vi "dimetix demo.vi"() -> ()   [LabVIEW 2016]
uses:
  message box enable.vi
  <vilib>/Instr/_visa.llb/VISA Configure Serial Port (Instr).vi
panel:
  in  "parity (0:none)":enum16{"None", "Odd", "Even", "Mark", "Space"}(ring)=enum."Even"
  in  "data bits (8) 2":u16=7 min=5 max=8 step=1
  in  "baud rate (9600)":u32=19200
  in  "laser read command":string="s0h"
  out "Numeric":dbl format="%#.3g"
  in  "RS232 \nTIMEOUT":i32=1000
  in  "SERIAL PORT 1":u16(ring) caption="SERIAL PORT" items=["COM1  (ASRL1  )", "COM3  (ASRL3  )", "COM15 (ASRL15  )", "", ""]
  out "READ BUFFER":string
  out "RTN CNT":u32
  out "ERROR WARN":bool caption="ERROR"
  in  "READ":bool
  in  "stop vi":bool
  in  "joint cluster PIPE01":T1(array[cluster]) {"length" format="%.2f"}
  in  "step 1\ninitalize serial":bool
  out "command sent":string="s0c\r\n"
  out "after substring":string="00001117\r\n"
  out "error out":errorcluster
  in  "DEFAULT":T2={"version"="v 1.0.1", "digitally download dir"=path "C:/Documents and Settings/All Users/Application Data/digitally/data", "data Xport path"=path "C:/Program Files/Unitronics/Unitronics DataXport/DataXport.exe", "HTML Save Path"=path "C:/Documents and Settings/All Users/Application Data/digitally/data", "UNIT LABEL"="FEET / TENTHS", "Company name"="Laser-View Technologies"}
  out "FILE SAVED ONCE":bool
  in  "INPUT CLUSTER":T3={"READ DIRECTION"=TRUE, "MEASUREMENT SOURCE"=0, "GROUP ANALYSIS METHOD"=0, "units"=2, "SERIAL PORT 1"=0, "SERIAL PORT 2"=1, "SERIAL PORT 3"=0, "GROUP SIZE"=1, "OFFSET- 2 laser"=0.0, "ACTUAL MEAUSURE"=0.0, "MEASURE SPEED"=2, "DISTANCE DELTA \nFOR FAST MODE (mm)"=1.0, "laser 1 OFFSET"=1.0, "laser 2 OFFSET"=0.0, "ENABLE SENSOR A"=TRUE, "ENABLE SENSOR B"=TRUE, "ENABLE SENSOR C"=TRUE, "PORT TIMEOUT (msec)"=300, "PASSWORD"="", "ENABLE ON-SCREEN\nKEYBOARD"=TRUE, "version"="", "BUFER LENGTH"=100, "TRIGGER DELAY (msec)"=100, "DATA LOG  FILE DIR"=path "C:/Documents and Settings/All Users/Application Data/PMS200", "MEASUREMENT TYPE"=0, "ENABLE DATA LOG"=FALSE, " LIMITS SENSOR 1"={"Upper tol"=4.3, "Lower tol"=0.0, "STATUS"=FALSE, "Boolean"=FALSE}, " LIMITS SENSOR 2"={"Upper tol"=0.0, "Lower tol"=0.0, "STATUS"=FALSE, "Boolean"=FALSE}, " CALC LIMITS"={"Upper tol"=0.0, "Lower tol"=0.0, "STATUS"=FALSE, "Boolean"=FALSE}, "LASER 2\n ENABLE"=FALSE, "LASER 1 \nENABLE"=TRUE, "BAUD RATE"=1, "PARITY"=2, "DATA BITS"=0, "TRIGGER OPERATION"=0, "TRIGGER LENGTH (sec)"=15.0, "BUFFER METHOD"=0, "DATA LOG METHOD"=0, "LASER 2"=TRUE, "LASER 1"=TRUE, "ACTUAL LASER 2"=0.0, "ACTUAL LASER 1"=0.0, "TWO LASER\n CALIBRATE"=0.0, "OFFSET- TWO LASER 2"=5.0, "Part identification"="100", "JOB ID"="FDFDF", "Operator"="5.5", "Notes"="5.5", "SIZE"="5.5", "WEIGHT"="100", "serial #"=101, "Company name"="BBBB", "LANGUAGE"=0, "LASER \nOFFSET THREADS OFF"=1.0, "LASER \nOFFSET THREADS ON"=1.0, "THREADS ON/OFF"=2, "OPERATION  "=0} {"OPERATION" items=["DRILL SITE- NO S/N", "PIPE YARD- INCLUDE S/N"]; "THREADS ON/OFF" items=["THREADS OFF", "THREADS ON"]; "LASER \nOFFSET THREADS ON" format="%.2f"; "LASER \nOFFSET THREADS OFF" format="%.2f"; "LANGUAGE" items=["ENGLISH", "SPANISH"]; "OFFSET- TWO LASER 2" format="%.2f"; "TWO LASER\n CALIBRATE" format="%.2f"; "ACTUAL LASER 1" format="%.2f"; "ACTUAL LASER 2" format="%.2f"; "DATA LOG METHOD" items=["CONTINUOUS", "TRIGGER SINGLE SHOT", "TRIGGER START/STOP"]; "BUFFER METHOD" items=["BUFFER IN MEMORY", "WRITE IMMEDIATELY"]; "TRIGGER LENGTH (sec)" format="%.1f"; "TRIGGER OPERATION" items=["CLICK START/STOP", "TIMED"]; "DATA BITS" items=["7 (LASER FACTORY DEFAULT", "8", "EVEN"]; "PARITY" items=["NONE", "ODD", "EVEN"]; "BAUD RATE" items=["9600", "19200", "38400", "57600", "115200"]; "CALC LIMITS"."Lower tol" format="%.3f"; "CALC LIMITS"."Upper tol" format="%.3f"; "LIMITS SENSOR 2"."Lower tol" format="%.3f"; "LIMITS SENSOR 2"."Upper tol" format="%.3f"; "LIMITS SENSOR 1"."Lower tol" format="%.3f"; "LIMITS SENSOR 1"."Upper tol" format="%.3f"; "MEASUREMENT TYPE" items=["DISTANCE ", "DIMENSION- SINGLE LASER", "DIMENSION- TWO LASERS DIFFERENTIAL", "DISTANCE DELTA- TWO LASERS"]; "laser 2 OFFSET" format="%.2f"; "laser 1 OFFSET" format="%.2f"; "DISTANCE DELTA \nFOR FAST MODE (mm)" format="%.2f"; "MEASURE SPEED" items=["STANDARD", "FAST"]; "ACTUAL MEAUSURE" format="%.2f"; "OFFSET- 2 laser" format="%.2f"; "GROUP SIZE" min=1; "SERIAL PORT 3" items=["COM1  (ASRL1  )", "COM4 (ASRL4  )", "COM8  (ASRL8  )", "COM9  (ASRL9  )", "", "", ""]; "SERIAL PORT 2" items=["COM1  (ASRL1  )", "COM4 (ASRL4  )", "COM8  (ASRL8  )", "COM9  (ASRL9  )", "", "", ""]; "SERIAL PORT 1" items=["COM1  (ASRL1  )", "COM4 (ASRL4  )", "COM8  (ASRL8  )", "COM9  (ASRL9  )", "", "", ""]; "units" items=["mm", "inch"]; "GROUP ANALYSIS METHOD" items=["mean", "median"]; "MEASUREMENT SOURCE" items=["LIVE", "EMULATE"]}
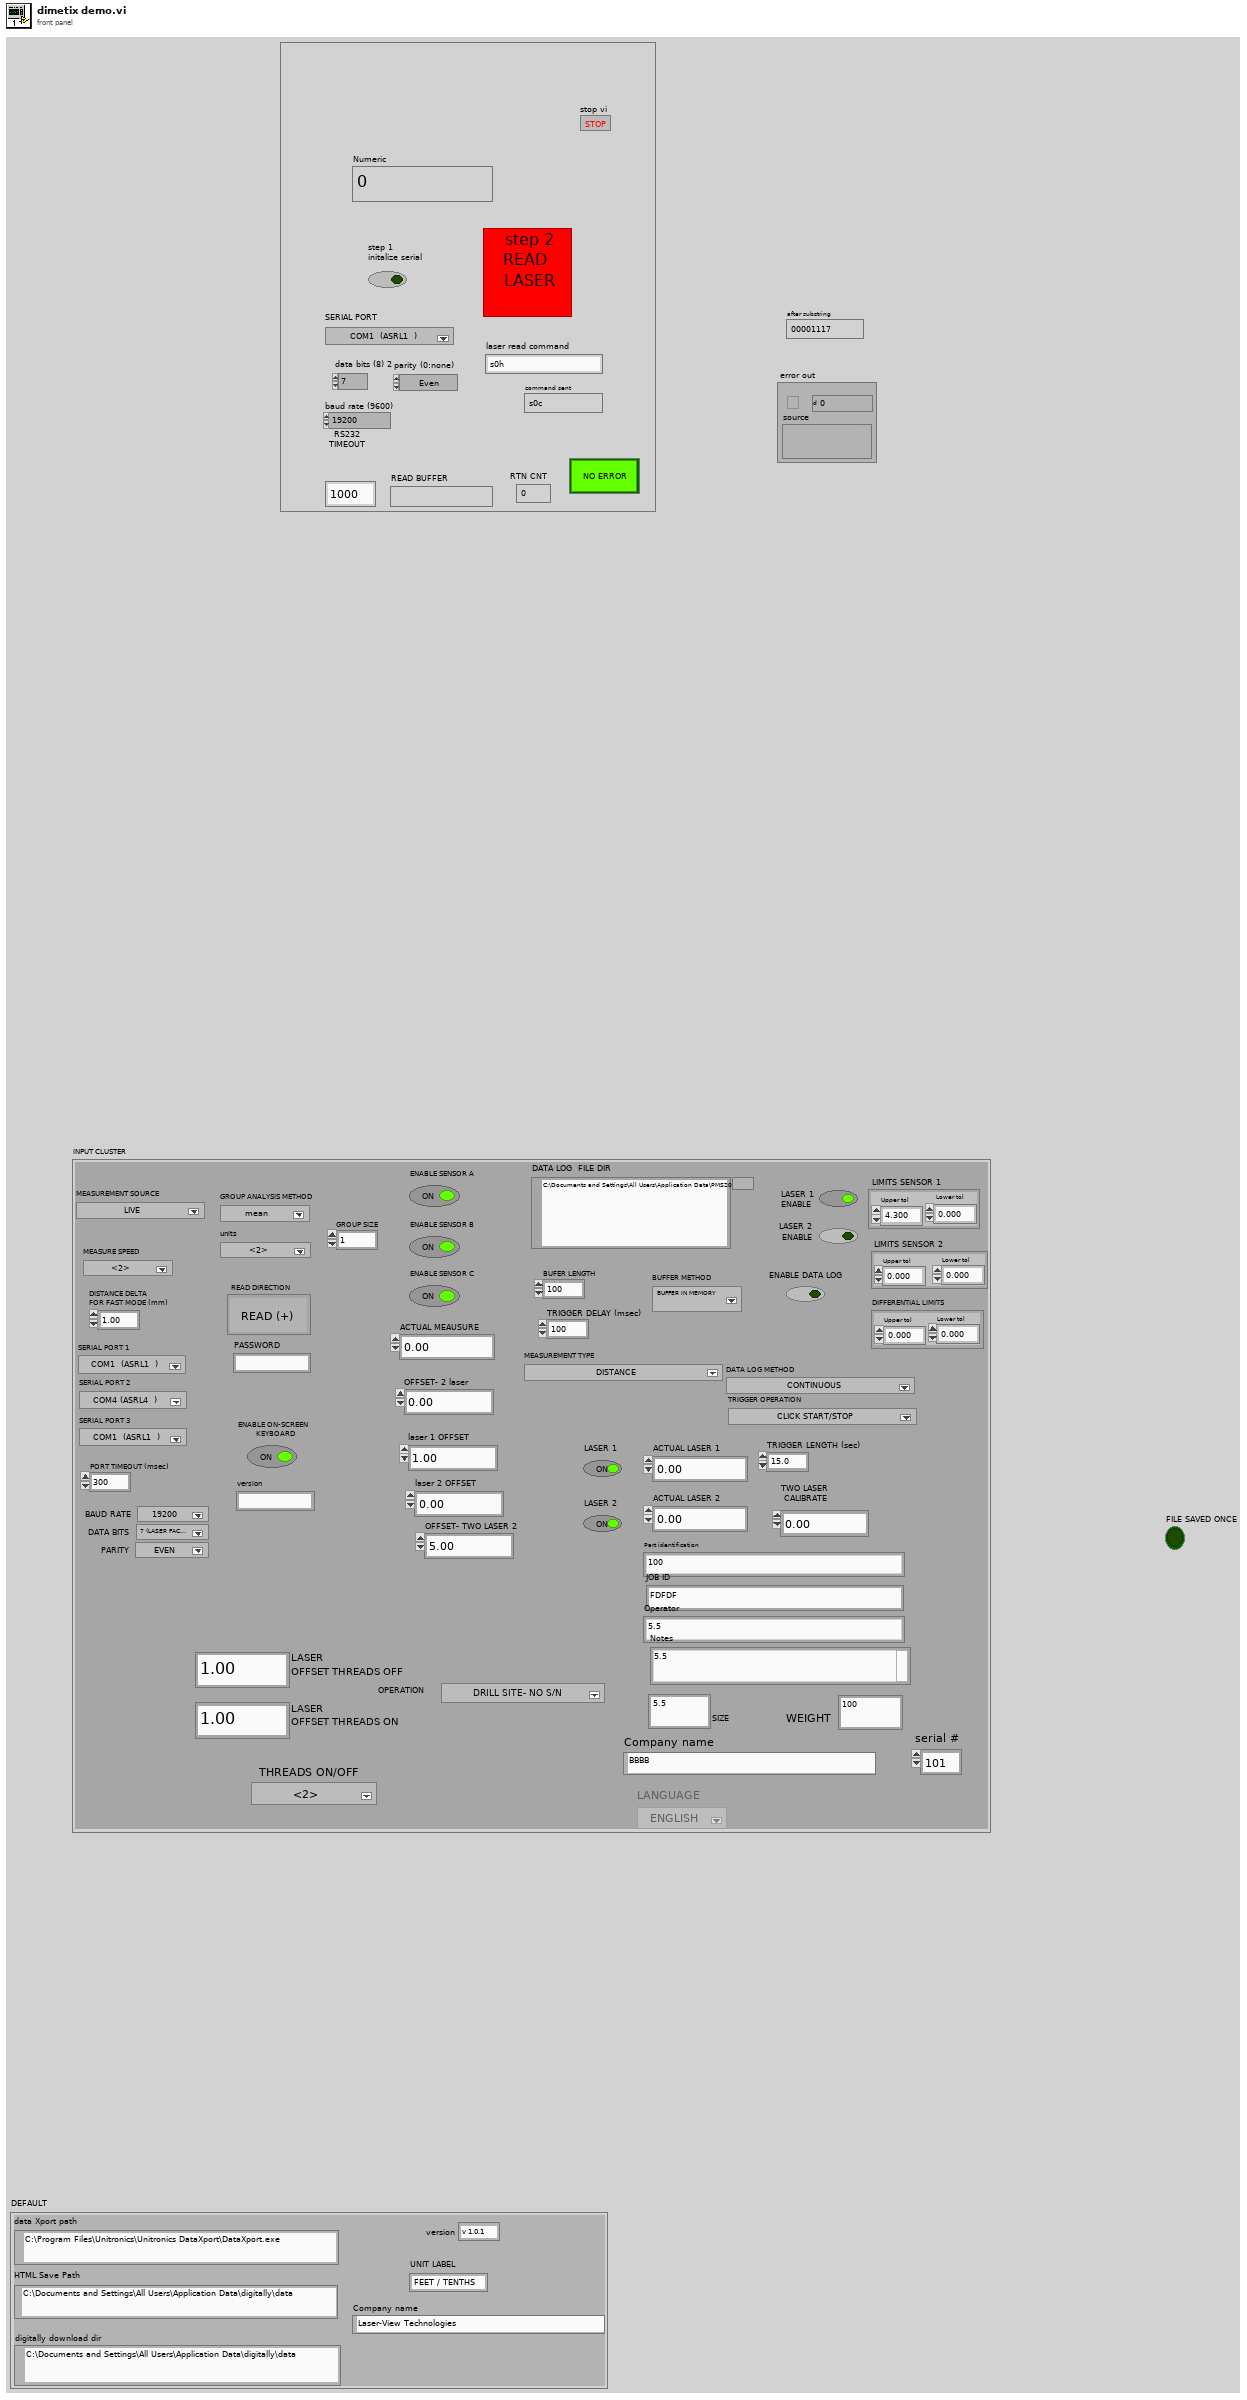
[diagram p1: front panel]
types:
  T1 = cluster{"joint":i32, "length":dbl, "s/n":string}[]
  T2 = cluster{"version":string, "digitally download dir":path, "data Xport path":path, "HTML Save Path":path, "UNIT LABEL":string, "Company name":string}
  T3 = cluster{"READ DIRECTION":bool, "MEASUREMENT SOURCE":u16, "GROUP ANALYSIS METHOD":u16, "units":u16, "SERIAL PORT 1":u16, "SERIAL PORT 2":u16, "SERIAL PORT 3":u16, "GROUP SIZE":i32, "OFFSET- 2 laser":dbl, "ACTUAL MEAUSURE":dbl, "MEASURE SPEED":u16, "DISTANCE DELTA \nFOR FAST MODE (mm)":dbl, "laser 1 OFFSET":dbl, "laser 2 OFFSET":dbl, "ENABLE SENSOR A":bool, "ENABLE SENSOR B":bool, "ENABLE SENSOR C":bool, "PORT TIMEOUT (msec)":i32, "PASSWORD":string, "ENABLE ON-SCREEN\nKEYBOARD":bool, "version":string, "BUFER LENGTH":i32, "TRIGGER DELAY (msec)":i32, "DATA LOG  FILE DIR":path, "MEASUREMENT TYPE":u16, "ENABLE DATA LOG":bool, " LIMITS SENSOR 1":cluster{"Upper tol":dbl, "Lower tol":dbl, "STATUS":bool, "Boolean":bool}, " LIMITS SENSOR 2":cluster{"Upper tol":dbl, "Lower tol":dbl, "STATUS":bool, "Boolean":bool}, " CALC LIMITS":cluster{"Upper tol":dbl, "Lower tol":dbl, "STATUS":bool, "Boolean":bool}, "LASER 2\n ENABLE":bool, "LASER 1 \nENABLE":bool, "BAUD RATE":u16, "PARITY":u16, "DATA BITS":u16, "TRIGGER OPERATION":u16, "TRIGGER LENGTH (sec)":dbl, "BUFFER METHOD":u16, "DATA LOG METHOD":u16, "LASER 2":bool, "LASER 1":bool, "ACTUAL LASER 2":dbl, "ACTUAL LASER 1":dbl, "TWO LASER\n CALIBRATE":dbl, "OFFSET- TWO LASER 2":dbl, "Part identification":string, "JOB ID":string, "Operator":string, "Notes":string, "SIZE":string, "WEIGHT":string, "serial #":i32, "Company name":string, "LANGUAGE":u16, "LASER \nOFFSET THREADS OFF":dbl, "LASER \nOFFSET THREADS ON":dbl, "THREADS ON/OFF":u16, "OPERATION  ":u16}
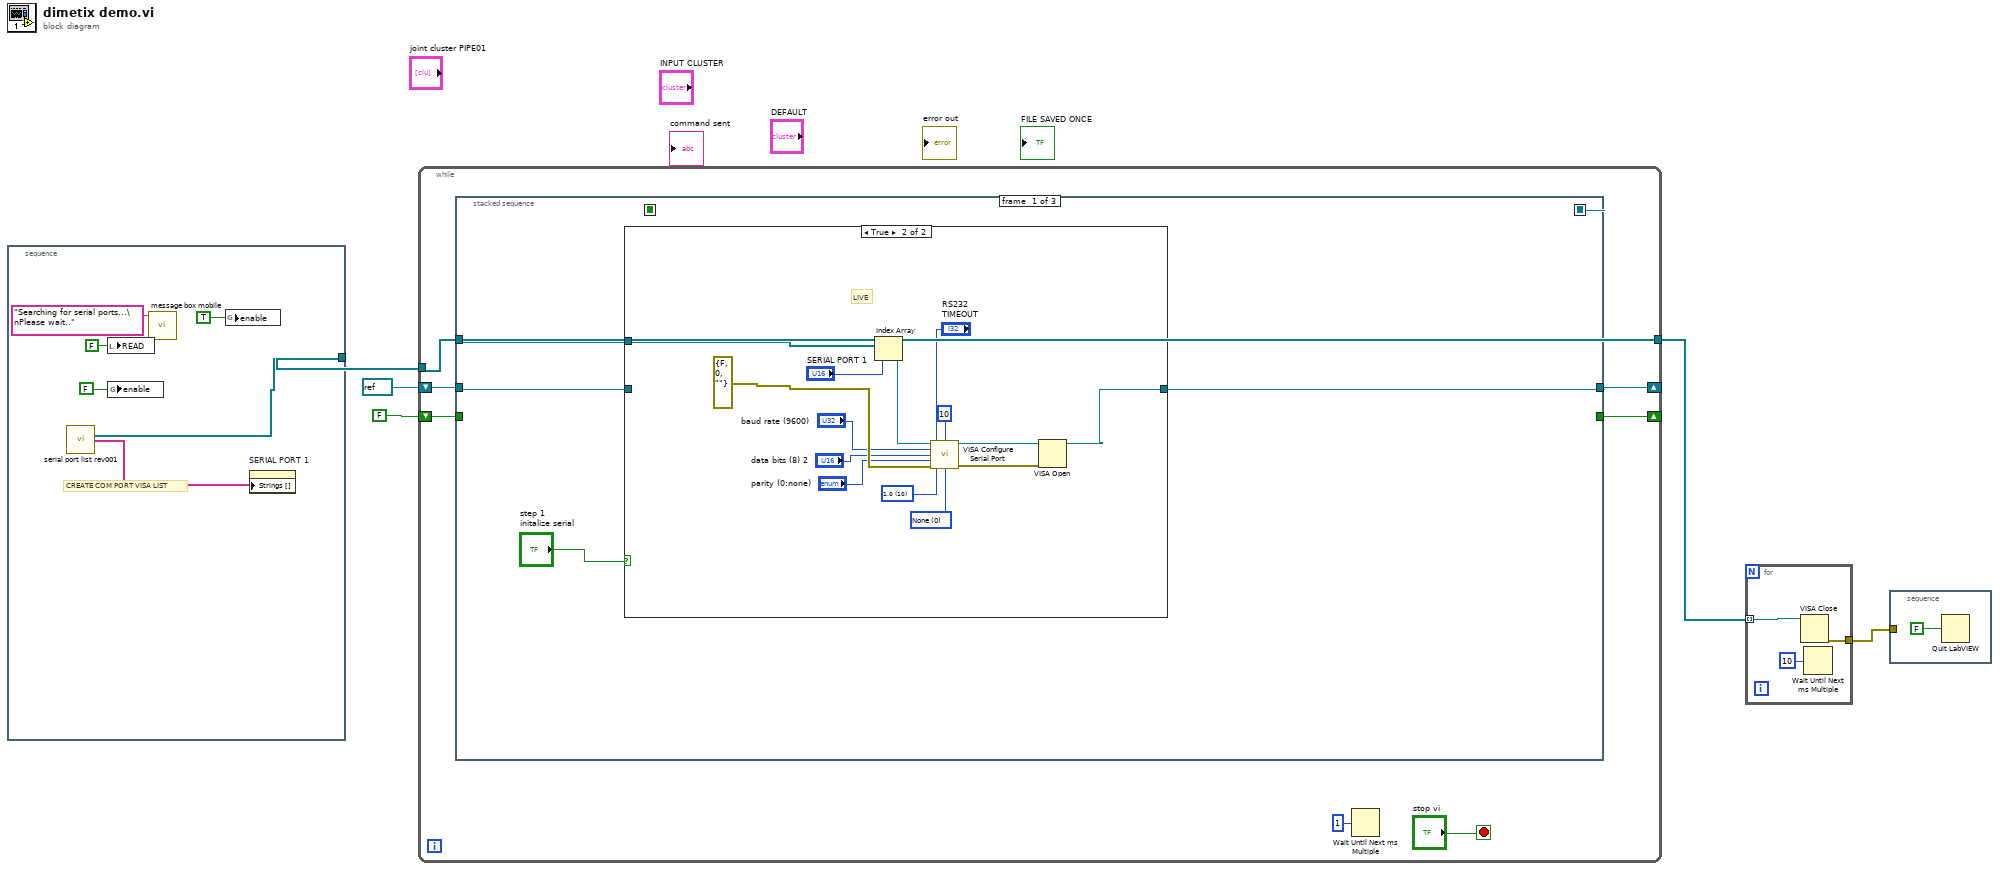
[diagram p0: block diagram]
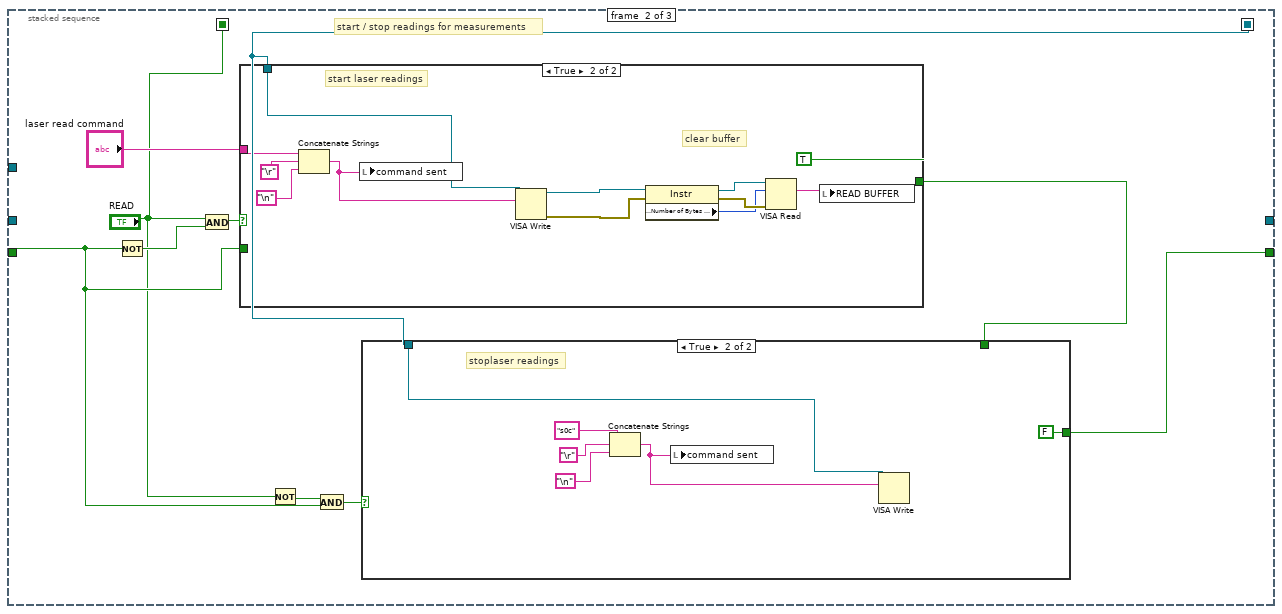
[diagram p3: hidden frame]
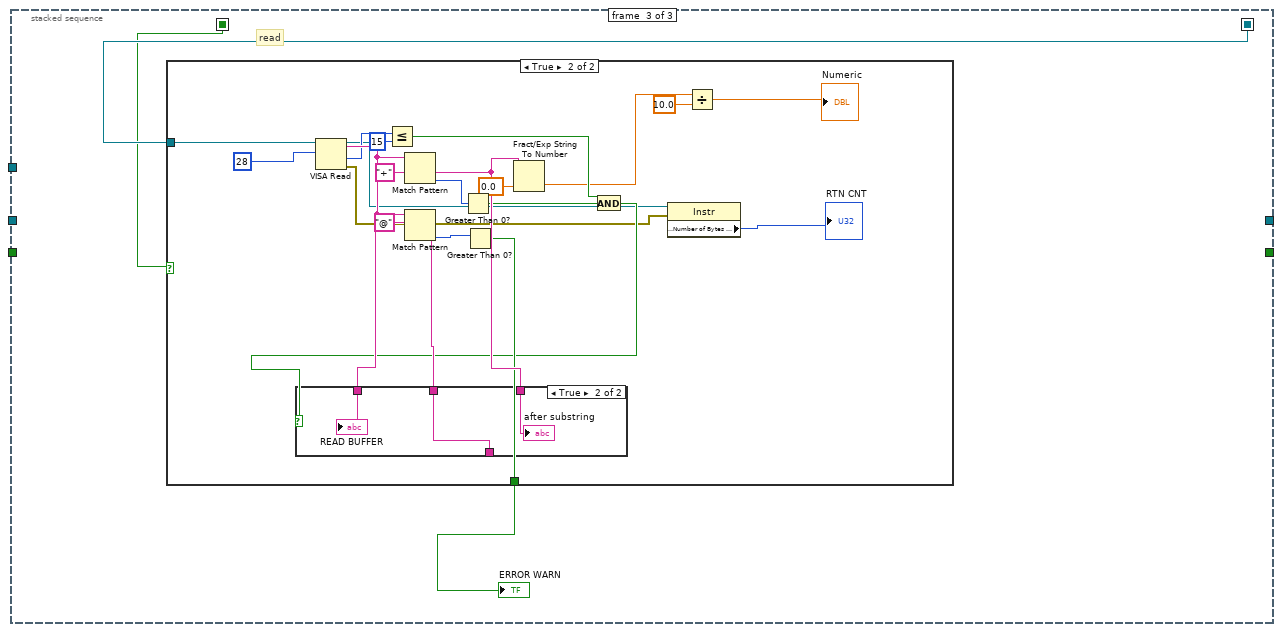
[diagram p6: hidden frame]
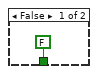
[diagram p7: hidden frame]
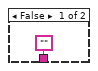
[diagram p8: hidden frame]
diagram:
  n1 = stacked-sequence {
    tunnel: [w11] -> w5
    frame #0 {
      # "CREATE COM PORT VISA LIST"
      n2 = call "serial port list rev001.vi"() -> ("I/O Array out"=w11:refnum<visa-resource-name>[], "com port names"=w10:string[])  [unwired: 14 out]
      n3 = local write "READ"(FALSE ("READ")) -> ()
      n4 = global write "message box enable.vi" "enable"(FALSE ("enable")) -> ()
      n5 = call "message box mobile.vi"("String"="Searching for serial ports...\nPlease wait..") -> ()  [unwired: 11 out]
      n6 = global write "message box enable.vi" "enable"(TRUE ("enable")) -> ()
      n7 = property on="SERIAL PORT 1" class="Ring (strict)"("Strings []"=w10) -> ()  [unwired: 2 in, 2 out]
    }
  }
  n8 = while {
    tunnel: w5 -> [w17]
    shift-right: [w18] -> _
    shift-left: refnum<visa-resource-name> refnum ("duplicate VISA resource name") -> [w16]
    tunnel: [w17] -> w3
    shift-right: [w13] -> _
    shift-left: FALSE -> [w14]
    stop <- "stop vi" stop-if-true
    n9 = stacked-sequence {
      seq-local: [w20 _ _] -> [_ w47 w69]
      seq-local: [_ "READ" _] -> [_ _ w68]
      tunnel: w17 -> [w22 _ _]
      tunnel: w16 -> [w21 _ _]
      tunnel: [w20 _ _] -> w18
      tunnel: w14 -> [_ w40 _]
      tunnel: [_ w41 _] -> w13
      frame #0 {
        n10 = case shown="True" "step 1\ninitalize serial" {
          tunnel: w22 -> [_ w37]
          tunnel: w21 -> [w23 _]
          tunnel: [w23 w36] -> w20
          frame False {
          }
          frame True {
            w29 = u16 0 items=["None", "XON/XOFF", "RTS/CTS", "XON/XOFF & RTS/CTS", "DTR/DSR", "XON/XOFF & DTR/DSR"] ("flow control (0:none)")
            w30 = u16 10 items=["1.0"=10, "1.5"=15, "2.0"=20] ("stop bits (10: 1 bit)")
            # "LIVE"
            n11 = Index Array(array=w37, index="SERIAL PORT 1") -> (element=w33:refnum<visa-resource-name>)
            n12 = call-poly "VISA Configure Serial Port"("VISA resource name"=w33, "timeout (10sec)"="RS232 \nTIMEOUT", "termination char\n(0xA = '\\n' = LF)"=u8 10 ("termination char\n(0xA = '\\n' = LF)"), "baud rate (9600)"="baud rate (9600)", "data bits (8)"="data bits (8) 2", "parity (0:none)"="parity (0:none)", "error in (no error)"=errorcluster {"status"=FALSE, "code"=0, "source"=""}, "stop bits (10: 1 bit)"=w30, "flow control (0:none)"=w29) -> ("VISA resource name out"=w27:refnum<visa-resource-name>, "error out"=w28:errorcluster)  [unwired: 5 out]
            n13 = VISA Open(error in (no error)=w28, VISA resource name=w27) -> (VISA resource name=w36:refnum<visa-resource-name>)  [unwired: 3 in, 1 out]
          }
        }
      }
      frame #1 {
        # "start / stop readings for measurements"
        n14 = Not(x=w40) -> (.not. x?=w45:bool)
        n15 = And(x="READ", y=w45) -> (x .and. y?=w38:bool)
        n16 = case shown="True" w38 {
          tunnel: w47 -> [_ w65]
          tunnel: [w55 TRUE] -> w42
          tunnel: "laser read command" -> [_ w57]
          tunnel: w40 -> [w55 _]
          frame False {
          }
          frame True {
            # "clear buffer"
            # "start laser readings"
            n17 = Concatenate Strings(w57, "\r", "\n") -> (w67:string)
            n18 = local write "command sent"(w67) -> ()
            n19 = VISA Write(VISA resource name=w65, write buffer=w67) -> (VISA resource name out=w63:refnum<visa-resource-name>, error out=w62:errorcluster)  [unwired: 1 in, 1 out]
            n20 = property class="Instr"(reference=w63, error in=w62) -> (reference out=w59:refnum<visa-resource-name>, error out=w61:errorcluster, "Serial Settings:Number of Bytes at Serial Port"=w60:u32)
            n21 = VISA Read(VISA resource name=w59, byte count=w60, error in (no error)=w61) -> (read buffer=w58:string)  [unwired: 3 out]
            n22 = local write "READ BUFFER"(w58) -> ()
          }
        }
        n23 = Not(x="READ") -> (.not. x?=w43:bool)
        n24 = And(x=w43, y=w40) -> (x .and. y?=w44:bool)
        n25 = case shown="True" w44 {
          tunnel: w47 -> [_ w50]
          tunnel: w42 -> [w48 _]
          tunnel: [w48 FALSE] -> w41
          frame False {
          }
          frame True {
            # "stoplaser readings"
            n26 = Concatenate Strings("s0c" ("write buffer (\"\")"), "\r", "\n") -> (w54:string)
            n27 = local write "command sent"(w54) -> ()
            n28 = VISA Write(VISA resource name=w50, write buffer=w54) -> ()  [unwired: 1 in, 3 out]
          }
        }
      }
      frame #2 {
        # "read"
        n29 = case shown="True" w68 {
          tunnel: [FALSE w89] -> w70
          tunnel: w69 -> [_ w76]
          frame False {
          }
          frame True {
            n30 = VISA Read(VISA resource name=w76, byte count=28) -> (VISA resource name out=w78:refnum<visa-resource-name>, read buffer=w93:string, return count=w82:u32, error out=w75:errorcluster)  [unwired: 1 in]
            n31 = Less Or Equal?(x=w82, y=u32 15) -> (x <= y?=w79:bool)
            n32 = Match Pattern(string=w93, regular expression="+") -> (after substring=w90:string, offset past match=w86:i32)  [unwired: 3 out]
            n33 = Match Pattern(string=w93, regular expression="@") -> (after substring=w92:string, offset past match=w83:i32)  [unwired: 3 out]
            n34 = Greater Than 0?(x=w86) -> (x > 0?=w80:bool)
            n35 = Greater Than 0?(x=w83) -> (x > 0?=w89:bool)
            n36 = Fract/Exp String To Number(string=w90, default (0 dbl)=0.0) -> (number=w74:dbl)  [unwired: 1 in, 2 out]
            n37 = And(x=w79, y=w80) -> (x .and. y?=w88:bool)
            n38 = case shown="True" w88 {
              tunnel: w93 -> [_ w97]
              tunnel: w90 -> [_ w96]
              tunnel: ["" w95] -> _
              tunnel: w92 -> [_ w95]
              frame False {
              }
              frame True {
                "READ BUFFER" <- w97
                "after substring" <- w96
              }
            }
            n39 = property class="Instr"(reference=w78, error in=w75) -> ("Serial Settings:Number of Bytes at Serial Port"=→"RTN CNT":u32)  [unwired: 2 out]
            n40 = Divide(x=w74, y=10.0) -> (x/y=→"Numeric":dbl)
          }
        }
        "ERROR WARN" <- w70
      }
    }
    n41 = Wait Until Next ms Multiple(millisecond multiple=u32 1) -> ()  [unwired: 1 out]
  }
  n42 = for {
    tunnel: w3 -> [w100] mode=indexing
    tunnel: [w98] -> w2
    n43 = VISA Close(VISA resource name=w100) -> (error out=w98:errorcluster)  [unwired: 1 in]
    n44 = Wait Until Next ms Multiple(millisecond multiple=u32 10) -> ()  [unwired: 1 out]
  }
  n45 = stacked-sequence {
    tunnel: w2 -> [_]
    frame #0 {
      n46 = Quit LabVIEW(quit? (T)=FALSE) -> ()
    }
  }
